vi "ATM Controller.vi"(8 "error in (no error)":errorcluster, 11 "View Model":T1) -> (0 "error out":errorcluster)   [LabVIEW 2017]
doc: "A software component that monitors and controls the transactions by interacting with other processes."
uses:
  View Model/Controls/View Model.ctl
  View Model/Controls/Shared Model.ctl
  Error Handler/Controls/Error Model.ctl
  Error Handler/Controls/Error Data.ctl
  Error Handler/Controls/Error Type.ctl
  Error Handler/Controls/Error Source.ctl
  Configuration/Controls/Config Model.ctl
  Configuration/Controls/Config CMD.ctl
  Configuration/Controls/Config Command.ctl
  Controls/Controller Model.ctl
  Controls/Controller Overhead.ctl
  Controls/Controller Transaction.ctl
  Controls/Controller State.ctl
  Configuration/Controls/Config Data Record.ctl
  Timing/Controls/Timer CMD.ctl
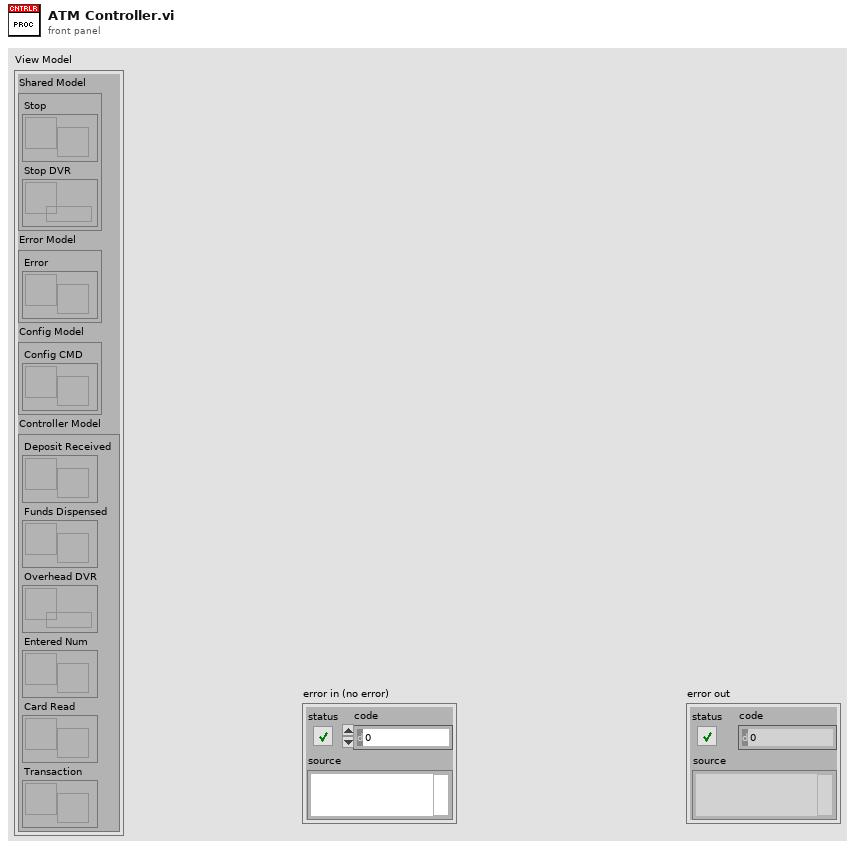
[diagram p1: front panel]
types:
  T1 = typedef "View Model.ctl" = cluster{"Shared Model":T2, "Error Model":T3, "Config Model":T4, "Controller Model":T5}
  T2 = typedef "Shared Model.ctl" = cluster{"Stop":refnum<user-event>, "Stop DVR":refnum<data-value>}
  T3 = typedef "Error Model.ctl" = cluster{"Error":refnum<user-event>}
  T4 = typedef "Config Model.ctl" = cluster{"Config CMD":refnum<user-event>}
  T5 = typedef "Controller Model.ctl" = cluster{"Deposit Received":refnum<user-event>, "Funds Dispensed":refnum<user-event>, "Overhead DVR":refnum<data-value>, "Entered Num":refnum<user-event>, "Card Read":refnum<user-event>, "Transaction":refnum<user-event>}
  T6 = typedef "Config Command.ctl" = enum16{"Read", "Search", "Update"}
  T7 = typedef "Timer CMD.ctl" = enum16{"Start", "Restart", "Get Time", "Pause", "UnPause"}
  T8 = typedef "Controller State.ctl" = enum16{"Idle", "Initial", "Login", "Balance Inquiry", "Deposit", "Withdrawal", "Fast Cash", "Terminate"}
  T9 = typedef "Controller Transaction.ctl" = enum16{"Balance Inquiry", "Deposit", "Withdrawal", "Fast Cash", "New Transaction", "Terminate Session"}
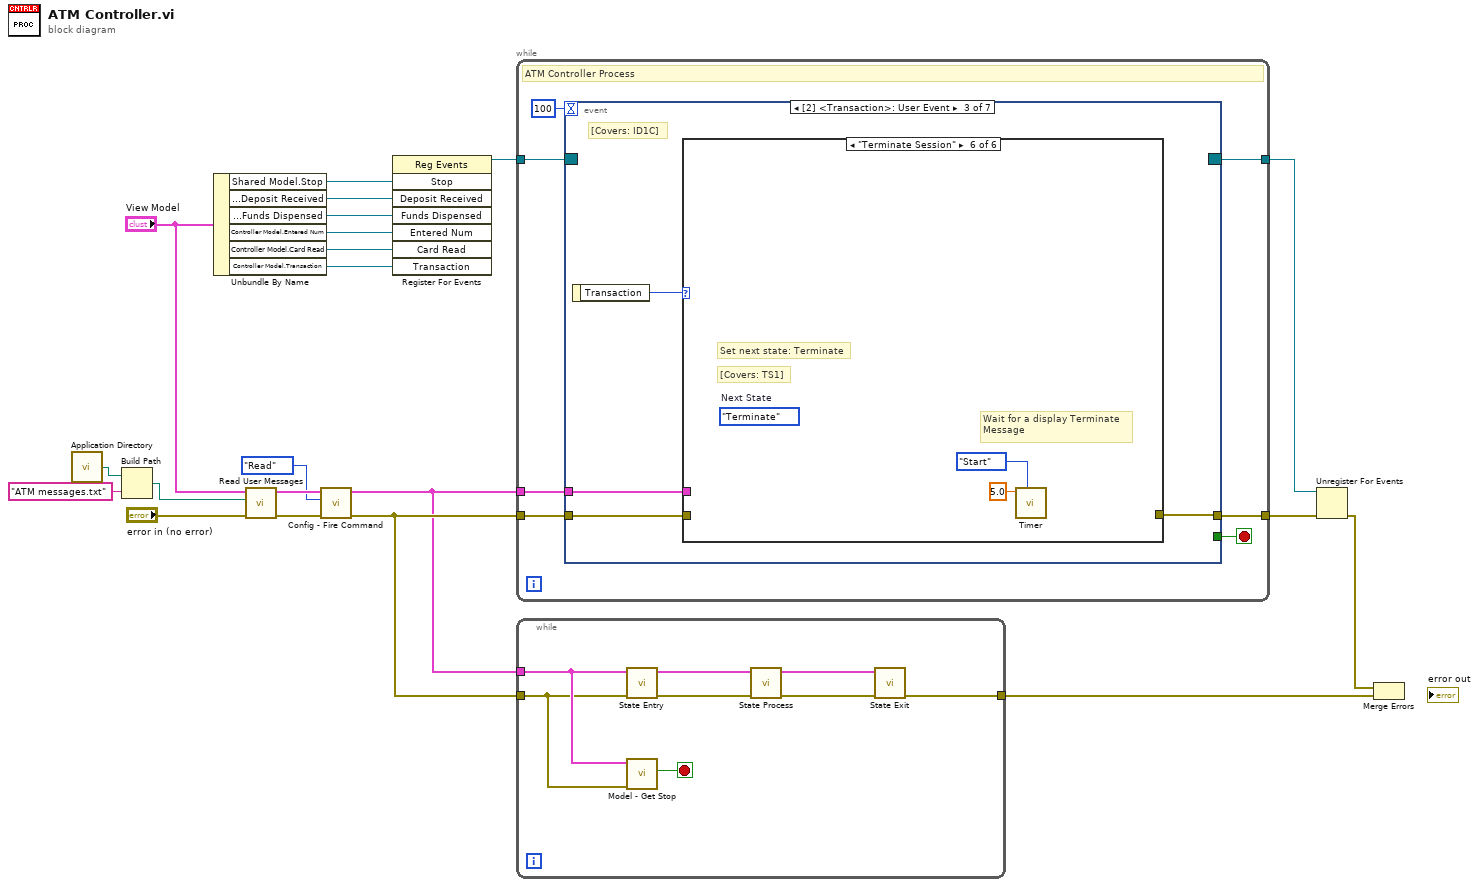
[diagram p0: block diagram]
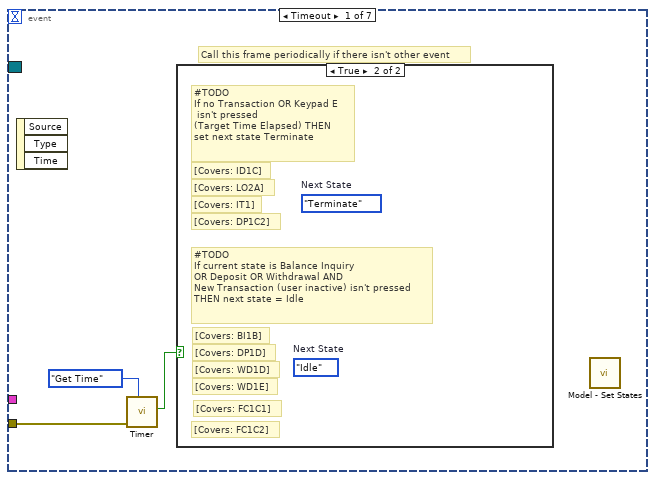
[diagram p2: hidden frame]
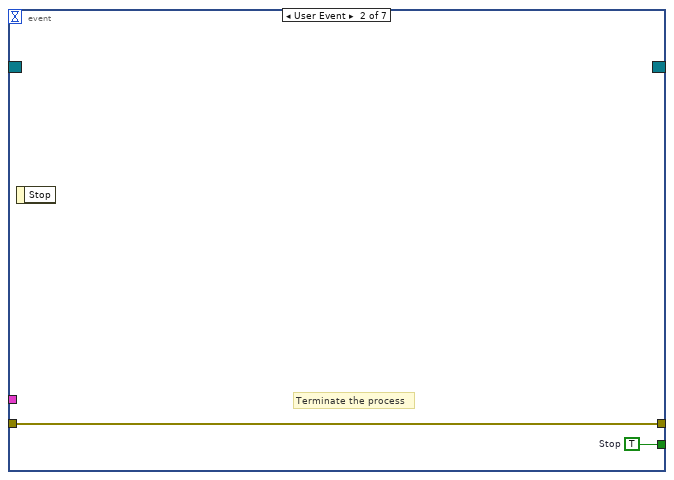
[diagram p4: hidden frame]
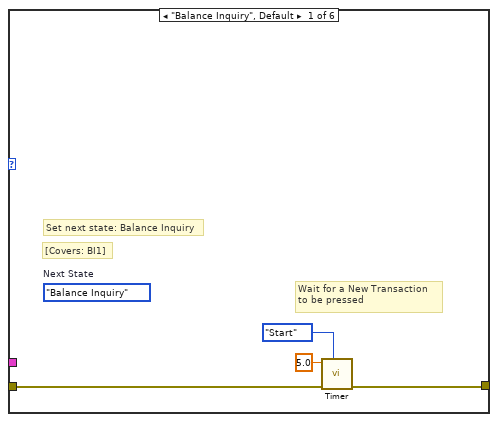
[diagram p5: hidden frame]
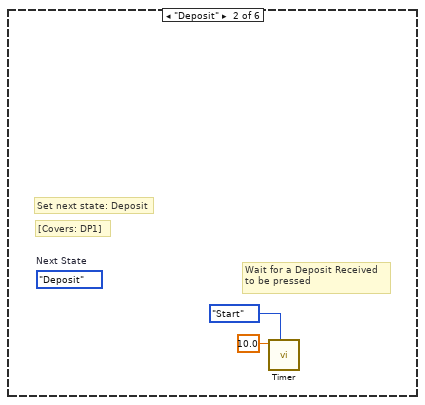
[diagram p6: hidden frame]
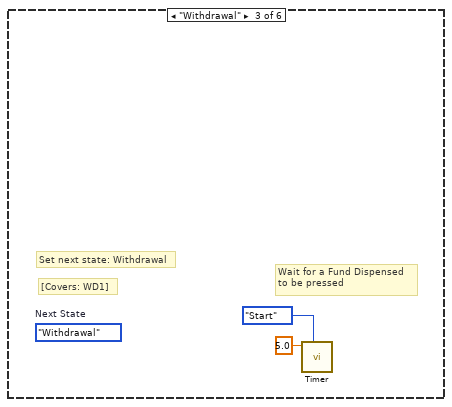
[diagram p7: hidden frame]
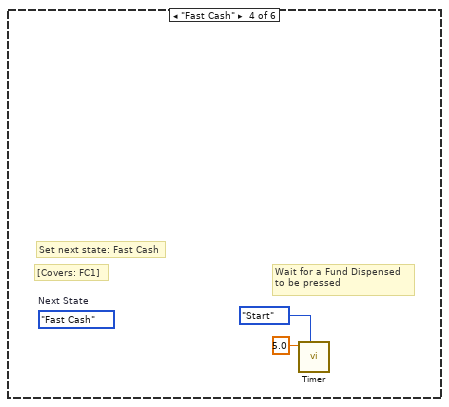
[diagram p8: hidden frame]
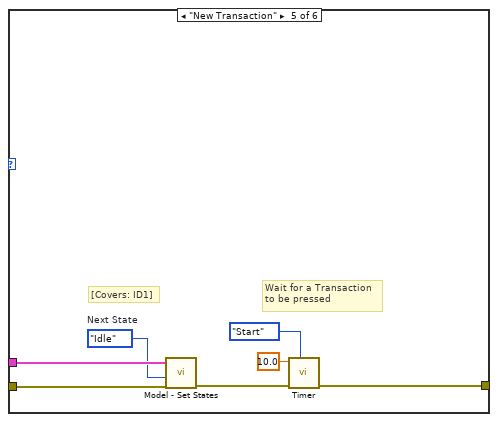
[diagram p9: hidden frame]
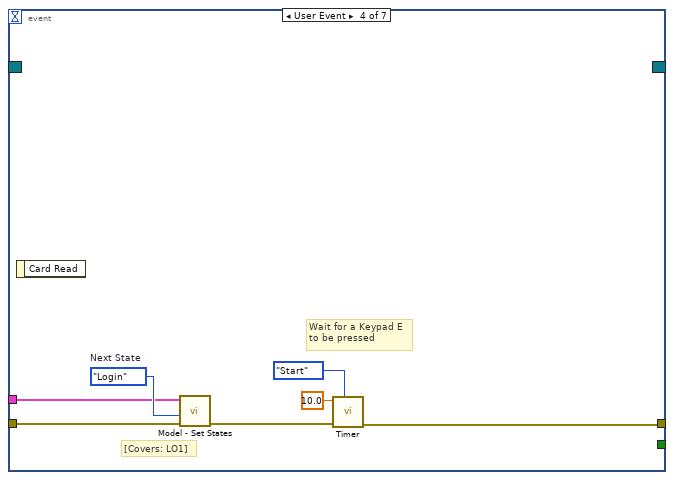
[diagram p10: hidden frame]
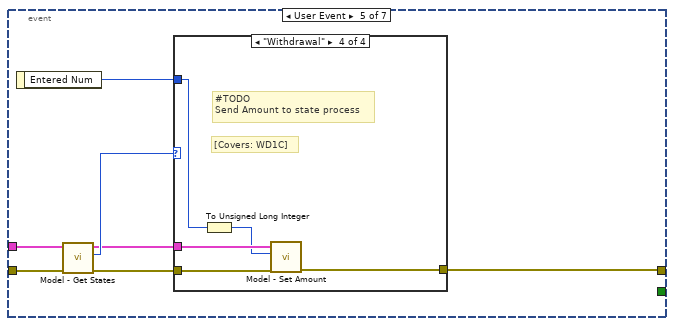
[diagram p11: hidden frame]
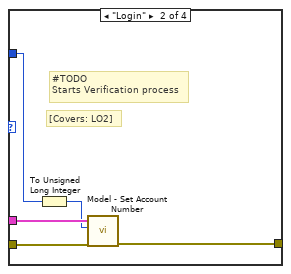
[diagram p13: hidden frame]
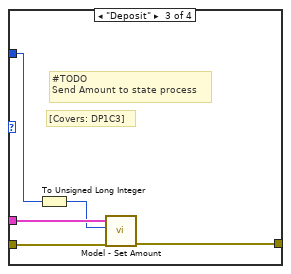
[diagram p14: hidden frame]
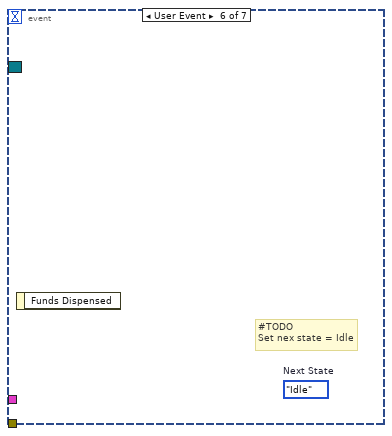
[diagram p15: hidden frame]
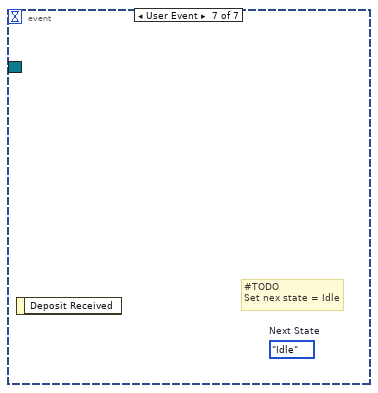
[diagram p16: hidden frame]
diagram:
  n1 = call <vilib>:"Application Directory.vi"() -> ("Application Directory"=w10:path)
  n2 = Build Path(base path=w10, name or relative path="ATM messages.txt") -> (appended path=w8:path)
  n3 = Unbundle By Name("View Model") -> ("Shared Model.Stop"=w21:refnum<user-event>, "Controller Model.Deposit Received"=w17:refnum<user-event>, "Controller Model.Funds Dispensed"=w16:refnum<user-event>, "Controller Model.Entered Num"=w15:refnum<user-event>, "Controller Model.Card Read"=w14:refnum<user-event>, "Controller Model.Transaction"=w13:refnum<user-event>)
  n4 = call "Read User Messages.vi"("error in (no error)"="error in (no error)", "Filepath"=w8, "View Model"="View Model") -> ("error out"=w6:errorcluster, "View Model"=w7:T1)  [unwired: 7 in]
  n5 = call "Config - Fire Command.vi"("error in (no error)"=w6, "CMD"=Config_Command."Read", "View Model"=w7) -> ("error out"=w5:errorcluster, "View Model"=w4:T1)  [unwired: 7 in]
  n6 = register-events(w21, w17, w16, w15, w14, w13) -> (reference out=w20:refnum<event-registration>)  [unwired: 2 in, 1 out]
  n7 = while {
    tunnel: w20 -> [w28]
    tunnel: [w27] -> w19
    tunnel: w5 -> [w26]
    tunnel: [w25] -> w18
    tunnel: w4 -> [w22]
    stop <- w23 stop-if-true
    # "ATM Controller Process"
    n8 = event shown="[2] <Transaction>: User Event" {
      selector: w28 -> [_ _ _ _ _ _ _]
      dyn-events: [_ _ _ _ _ _ _] -> w27
      timeout: 100 -> [_ _ _ _ _ _ _]
      tunnel: w26 -> [w31 w33 w35 w61 w70 _ _]
      tunnel: [_ w33 w34 w57 w64 _ _] -> w25
      tunnel: [_ w32 _ _ _ _ _] -> w23
      tunnel: w22 -> [_ _ w36 w62 w69 _ _]
      event Timeout {
        # "Call this frame periodically if there isn't other event"
        n9 = event-data() -> ()  [unwired: 1 in, 3 out]
        n10 = call "Timer.vi"("Timer CMD"=Timer_CMD."Get Time", "error in (no error)"=w31) -> ("Elapsed?"=w29:bool)  [unwired: 7 in, 2 out]
        n11 = case shown="True" w29 {
          frame False {
          }
          frame True {
            (unwired) Controller_State."Idle"  # Next State
            (unwired) Controller_State."Terminate"  # Next State
            # "[Covers: FC1C2]"
            # "[Covers: FC1C1]"
            # "[Covers: WD1E]"
            # "[Covers: WD1D]"
            # "[Covers: DP1D]"
            # "[Covers: DP1C2]"
            # "[Covers: IT1]"
            # "[Covers: BI1B]"
            # "#TODO\nIf current state is Balance Inquiry \nOR Deposit OR Withdrawal AND \nNew Transaction (user inactive) isn't pressed \nTHEN next state = Idle"
            # "[Covers: LO2A]"
            # "[Covers: ID1C]"
            # "#TODO\nIf no Transaction OR Keypad E\n isn't pressed \n(Target Time Elapsed) THEN\nset next state Terminate"
          }
        }
        n12 = call "Model - Set States.vi"() -> ()  [unwired: 10 in, 2 out]
      }
      event User Event {
        w32 = TRUE  # Stop
        # "Terminate the process"
        n13 = event-data() -> ()  [unwired: 1 in, 1 out]
      }
      event User Event {
        # "[Covers: ID1C]"
        n14 = event-data() -> ("Transaction"=w37:T9)  [unwired: 1 in]
        n15 = case shown="\"Terminate Session\"" w37 {
          tunnel: w36 -> [_ _ _ _ w53 _]
          tunnel: w35 -> [w39 _ _ _ w54 _]
          tunnel: [w38 _ _ _ w50 _] -> w34
          frame "Balance Inquiry", Default {
            (unwired) Controller_State."Balance Inquiry"  # Next State
            # "Wait for a New Transaction\nto be pressed"
            # "[Covers: BI1]"
            # "Set next state: Balance Inquiry"
            n16 = call "Timer.vi"("Timer CMD"=Timer_CMD."Start", "error in (no error)"=w39, "Target Time"=5.0) -> ("error out"=w38:errorcluster)  [unwired: 6 in, 2 out]
          }
          frame "Deposit" {
            (unwired) Controller_State."Deposit"  # Next State
            # "Wait for a Deposit Received\nto be pressed"
            # "[Covers: DP1]"
            # "Set next state: Deposit"
            n17 = call "Timer.vi"("Timer CMD"=Timer_CMD."Start", "Target Time"=10.0) -> ()  [unwired: 7 in, 3 out]
          }
          frame "Withdrawal" {
            (unwired) Controller_State."Withdrawal"  # Next State
            # "Wait for a Fund Dispensed\nto be pressed"
            # "[Covers: WD1]"
            # "Set next state: Withdrawal"
            n18 = call "Timer.vi"("Timer CMD"=Timer_CMD."Start", "Target Time"=5.0) -> ()  [unwired: 7 in, 3 out]
          }
          frame "Fast Cash" {
            (unwired) Controller_State."Fast Cash"  # Next State
            # "Wait for a Fund Dispensed\nto be pressed"
            # "[Covers: FC1]"
            # "Set next state: Fast Cash"
            n19 = call "Timer.vi"("Timer CMD"=Timer_CMD."Start", "Target Time"=5.0) -> ()  [unwired: 7 in, 3 out]
          }
          frame "New Transaction" {
            w52 = Controller_State."Idle"  # Next State
            # "Wait for a Transaction\nto be pressed"
            # "[Covers: ID1]"
            n20 = call "Model - Set States.vi"("error in (no error)"=w54, "Next State"=w52, "View Model"=w53) -> ("error out"=w51:errorcluster)  [unwired: 7 in, 1 out]
            n21 = call "Timer.vi"("Timer CMD"=Timer_CMD."Start", "error in (no error)"=w51, "Target Time"=10.0) -> ("error out"=w50:errorcluster)  [unwired: 6 in, 2 out]
          }
          frame "Terminate Session" {
            (unwired) Controller_State."Terminate"  # Next State
            # "Wait for a display Terminate\nMessage"
            # "[Covers: TS1]"
            # "Set next state: Terminate"
            n22 = call "Timer.vi"("Timer CMD"=Timer_CMD."Start", "Target Time"=5.0) -> ()  [unwired: 7 in, 3 out]
          }
        }
      }
      event User Event {
        w63 = Controller_State."Login"  # Next State
        # "Wait for a Keypad E\nto be pressed"
        # "[Covers: LO1]"
        n23 = event-data() -> ()  [unwired: 1 in, 1 out]
        n24 = call "Model - Set States.vi"("error in (no error)"=w61, "Next State"=w63, "View Model"=w62) -> ("error out"=w58:errorcluster)  [unwired: 7 in, 1 out]
        n25 = call "Timer.vi"("Timer CMD"=Timer_CMD."Start", "error in (no error)"=w58, "Target Time"=10.0) -> ("error out"=w57:errorcluster)  [unwired: 6 in, 2 out]
      }
      event User Event {
        n26 = event-data() -> ("Entered Num"=w67:i32)  [unwired: 1 in]
        n27 = call "Model - Get States.vi"("error in (no error)"=w70, "View Model"=w69) -> ("error out"=w65:errorcluster, "Current State"=w68:T8, "View Model"=w66:T1)  [unwired: 6 in, 1 out]
        n28 = case shown="\"Withdrawal\"" w68 {
          tunnel: w67 -> [_ w74 w81 w86]
          tunnel: w66 -> [_ w75 w80 w85]
          tunnel: w65 -> [w71 w76 w79 w84]
          tunnel: [w71 w72 w77 w82] -> w64
          frame Default {
          }
          frame "Login" {
            # "[Covers: LO2]"
            # "#TODO\nStarts Verification process"
            n29 = To Unsigned Long Integer(number=w74) -> (unsigned 32bit integer=w73:u32)
            n30 = call "Model - Set Account Number.vi"("error in (no error)"=w76, "Account Number"=w73, "View Model"=w75) -> ("error out"=w72:errorcluster)  [unwired: 7 in, 1 out]
          }
          frame "Deposit" {
            # "[Covers: DP1C3]"
            # "#TODO\nSend Amount to state process"
            n31 = To Unsigned Long Integer(number=w81) -> (unsigned 32bit integer=w78:u32)
            n32 = call "Model - Set Amount.vi"("error in (no error)"=w79, "Amount"=w78, "View Model"=w80) -> ("error out"=w77:errorcluster)  [unwired: 7 in, 1 out]
          }
          frame "Withdrawal" {
            # "#TODO\nSend Amount to state process"
            # "[Covers: WD1C]"
            n33 = To Unsigned Long Integer(number=w86) -> (unsigned 32bit integer=w83:u32)
            n34 = call "Model - Set Amount.vi"("error in (no error)"=w84, "Amount"=w83, "View Model"=w85) -> ("error out"=w82:errorcluster)  [unwired: 7 in, 1 out]
          }
        }
      }
      event User Event {
        (unwired) Controller_State."Idle"  # Next State
        # "#TODO\nSet nex state = Idle"
        n35 = event-data() -> ()  [unwired: 1 in, 1 out]
      }
      event User Event {
        (unwired) Controller_State."Idle"  # Next State
        # "#TODO\nSet nex state = Idle"
        n36 = event-data() -> ()  [unwired: 1 in, 1 out]
      }
    }
  }
  n37 = while {
    tunnel: w4 -> [w89]
    tunnel: w5 -> [w88]
    tunnel: [w90] -> w2
    stop <- w87 stop-if-true
    n38 = call "State Entry.vi"("error in (no error)"=w88, "View Model"=w89) -> ("error out"=w92:errorcluster, "View Model"=w94:T1)  [unwired: 8 in]
    n39 = call "Model - Get Stop.vi"("error in (no error)"=w88, "View Model"=w89) -> ("Stop"=w87:bool)  [unwired: 7 in, 2 out]
    n40 = call "State Process.vi"("error in (no error)"=w92, "View Model"=w94) -> ("error out"=w91:errorcluster, "View Model"=w93:T1)  [unwired: 8 in]
    n41 = call "State Exit.vi"("error in (no error)"=w91, "View Model"=w93) -> ("error out"=w90:errorcluster)  [unwired: 8 in, 1 out]
  }
  n42 = Unregister For Events(event registration refnum=w19, error in=w18) -> (error out=w1:errorcluster)
  n43 = Merge Errors(w1, w2) -> ()  [unwired: 1 out]
